vi "testDataPass_v2,1_vi1.vi"() -> ()   [LabVIEW 2014]
uses:
  testDataPass_v2,0_global1.vi
panel:
  in  "stop":bool
  in  "arrTF_write":bool[](array[boolean])
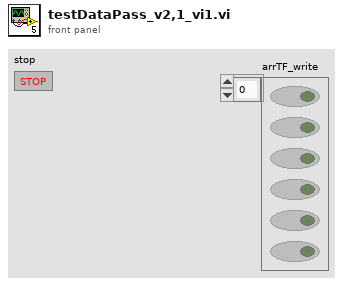
[diagram p1: front panel]
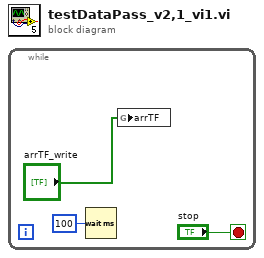
[diagram p0: block diagram]
diagram:
  n1 = while {
    stop <- "stop" stop-if-true
    n2 = Wait (ms)(milliseconds to wait=u32 100) -> ()  [unwired: 1 out]
    n3 = global write "testDataPass_v2,0_global1.vi" "arrTF"("arrTF_write") -> ()
  }
